vi "THERMOMETER using switch case.vi"() -> ()   [LabVIEW 2015]
panel:
  out "?":string
  out "Thermometer":dbl(slide) scale=0.0..120.0
  out "?":bool
  in  "?":string
  in  "?":bool
  out "Max Temp (F)":dbl
  in  "S5":dbl
  in  "S4":dbl
  in  "S3":dbl
  in  "S2":dbl
  in  "S1":dbl
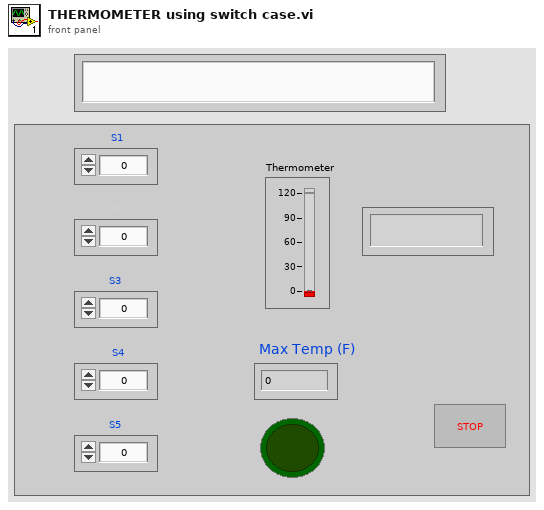
[diagram p1: front panel]
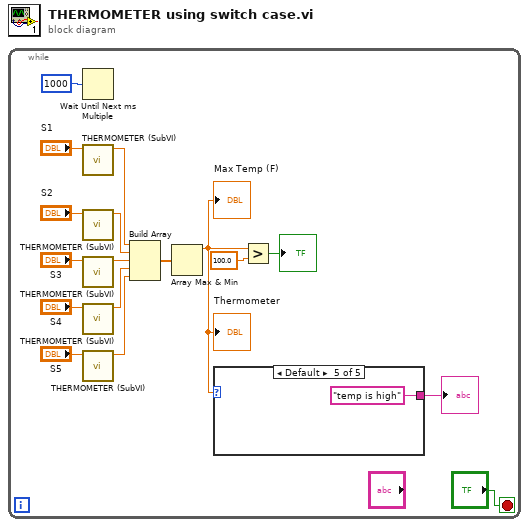
[diagram p0: block diagram]
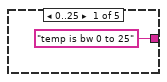
[diagram p2: hidden frame]
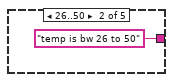
[diagram p3: hidden frame]
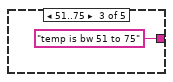
[diagram p4: hidden frame]
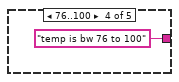
[diagram p5: hidden frame]
diagram:
  n1 = while {
    stop <- "?" stop-if-true
    n2 = Wait Until Next ms Multiple(millisecond multiple=u32 1000) -> ()  [unwired: 1 out]
    n3 = call "THERMOMETER (SubVI).vi"("Sensor 1"="S1") -> ("Numeric"=w10:dbl)  [unwired: 10 in]
    n4 = call "THERMOMETER (SubVI).vi"("Sensor 1"="S2") -> ("Numeric"=w9:dbl)  [unwired: 10 in]
    n5 = call "THERMOMETER (SubVI).vi"("Sensor 1"="S3") -> ("Numeric"=w8:dbl)  [unwired: 10 in]
    n6 = call "THERMOMETER (SubVI).vi"("Sensor 1"="S4") -> ("Numeric"=w7:dbl)  [unwired: 10 in]
    n7 = call "THERMOMETER (SubVI).vi"("Sensor 1"="S5") -> ("Numeric"=w6:dbl)  [unwired: 10 in]
    n8 = Build Array(w10, w9, w8, w7, w6) -> (w5:dbl[])
    n9 = Array Max & Min(array=w5) -> (max value=w1:dbl)  [unwired: 3 out]
    "Max Temp (F)" <- w1
    "Thermometer" <- w1
    n10 = case shown="Default" w1 {
      tunnel: ["temp is bw 0 to 25" "temp is bw 26 to 50" "temp is bw 51 to 75" "temp is bw 76 to 100" "temp is high"] -> w2
      frame 0..25 {
      }
      frame 26..50 {
      }
      frame 51..75 {
      }
      frame 76..100 {
      }
      frame Default {
      }
    }
    "?" <- w2
    n11 = Greater?(x=w1, y=100.0) -> (0:→"?":bool)
  }
